vi "_Enqueue CSMQ.vi"(8 "Error in":errorcluster caption="Error in (no error)", 10 "Data":T1, 11 "CSMQ in":T3) -> (0 "Error out":errorcluster, 1 "Target Busy Error":bool, 3 "CSMQ out":T3)   [LabVIEW 2014, in "Communicable State Machine.lvlib"]
uses:
  Communicable State Machine.lvlib
  _CSMQ.ctl
  Typedef/_Cross JKISM State Data.ctl
  Typedef/_CSM_MSG_TYPE.ctl
  Typedef/_Cross JKISM State Response.ctl
  Typedef/_CSM_MODE.ctl
  Typedef/_CSM Status Change Event Data.ctl
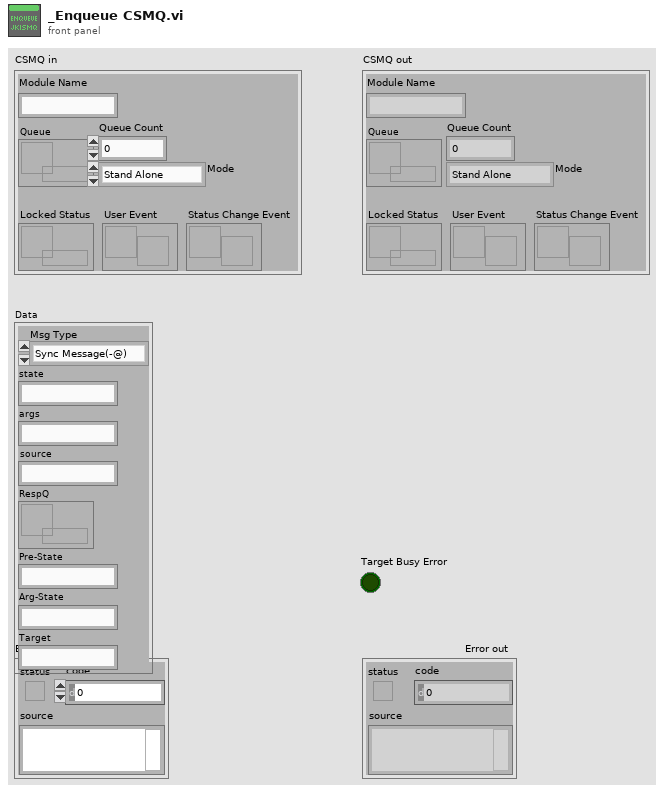
[diagram p1: front panel]
types:
  T1 = typedef "Communicable State Machine.lvlib/_Cross JKISM State Data.ctl" = cluster{"Msg Type":T2, "state":string, "args":string, "source":string, "RespQ":refnum<queue>, "Pre-State":string, "Arg-State":string, "Target":string}
  T2 = typedef "Communicable State Machine.lvlib/_CSM_MSG_TYPE.ctl" = enum16{"Sync Message(-@)", "Async Message(->)", "Async without Response(->|)", "Async Response", "Broadcast(-><status>)", "Broadcast(-><interrupt>)", "Request to Post Message", "Request to Post Message without Reply", "Request to Publish Status"}
  T3 = typedef "Communicable State Machine.lvlib/_CSMQ.ctl" = cluster{"Module Name":string, "Queue":refnum<queue>, "Locked Status":refnum<data-value>, "Mode":T4, "User Event":refnum<user-event>, "Queue Count":i32, "Status Change Event":refnum<user-event>}
  T4 = typedef "Communicable State Machine.lvlib/_CSM_MODE.ctl" = enum16{"Stand Alone", "JKISM", "Action Worker"}
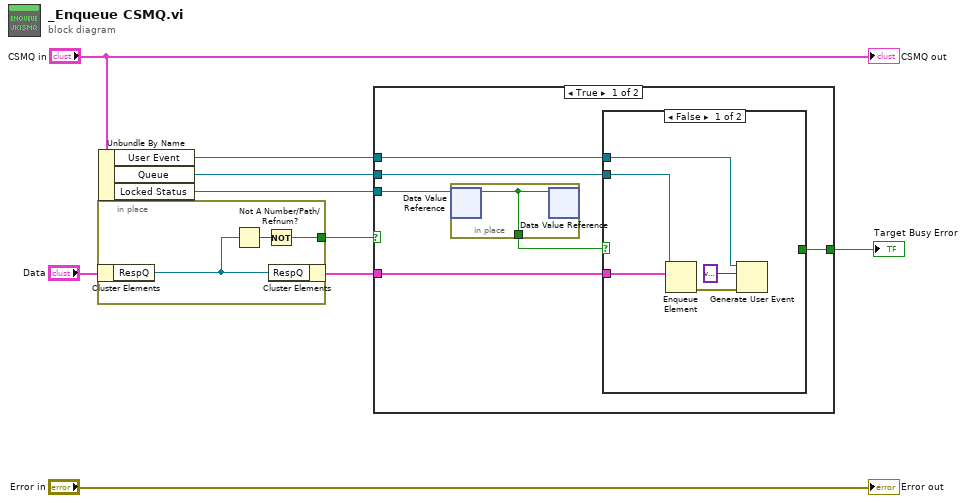
[diagram p0: block diagram]
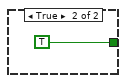
[diagram p2: hidden frame]
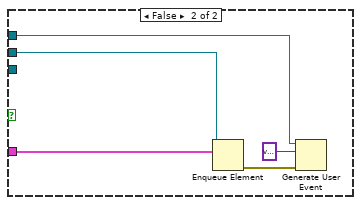
[diagram p3: hidden frame]
diagram:
  n1 = in-place {
    in-place-border: [w10] -> w5
    n2 = in-place-cluster #1("Data") -> ("RespQ"=w12:refnum<queue>)
    n3 = Not A Number/Path/Refnum?(number/path/refnum=w12) -> (NaN/Path/Refnum?=w11:bool)
    n4 = Not(x=w11) -> (.not. x?=w10:bool)
    n5 = in-place-cluster #1("RespQ"=w12) -> (w6:T1)
  }
  n6 = Unbundle By Name("CSMQ in") -> ("User Event"=w1:refnum<user-event>, "Queue"=w7:refnum<queue>, "Locked Status"=w4:refnum<data-value>)
  n7 = case shown="True" w5 {
    tunnel: w7 -> [w18 w30]
    tunnel: w6 -> [w17 w29]
    tunnel: w4 -> [w16 _]
    tunnel: [w14 _] -> w2
    tunnel: w1 -> [w13 w26]
    frame True {
      n8 = in-place {
        in-place-border: [w19] -> w15
        n9 = in-place-dvr #2(w16) -> (w19:bool)  [unwired: 1 out]
        n10 = in-place-dvr #2(w19) -> ()  [unwired: 2 out]
      }
      n11 = case shown="False" w15 {
        tunnel: w18 -> [w24 _]
        tunnel: w17 -> [w23 _]
        tunnel: [_ TRUE] -> w14
        tunnel: w13 -> [w21 _]
        frame False {
          n12 = Enqueue Element(queue=w24, element=w23) -> (error out=w22:errorcluster)  [unwired: 2 in, 2 out]
          n13 = Generate User Event(user event=w21, event data cluster=variant ("event data"), error in=w22) -> ()  [unwired: 1 in, 2 out]
        }
        frame True {
        }
      }
    }
    frame False {
      n14 = Enqueue Element(queue=w30, element=w29) -> (error out=w27:errorcluster)  [unwired: 2 in, 2 out]
      n15 = Generate User Event(user event=w26, event data cluster=variant ("event data"), error in=w27) -> ()  [unwired: 1 in, 2 out]
    }
  }
  "Target Busy Error" <- w2
  "Error out" <- "Error in"
  "CSMQ out" <- "CSMQ in"
